vi "GDSLvClass_OpenClass.vi"(1 "ClassToOpen":path, 5 "error in (no error)":errorcluster, 6 "Project/ApplicationRef(If empty, currect active project will be used)":variant) -> (14 "LVClass.Open":refnum<vi>, 19 "error out":errorcluster)   [LabVIEW 2020]
panel:
  in  "App Ref 2":refnum<vi>
  in  "App Refnum 2":refnum<vi>
  in  "Array 2":refnum<vi>[](array[refnum])
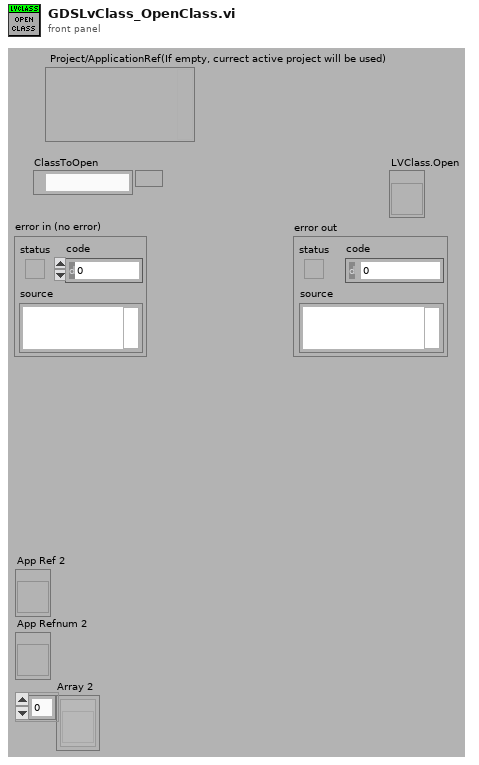
[diagram p1: front panel]
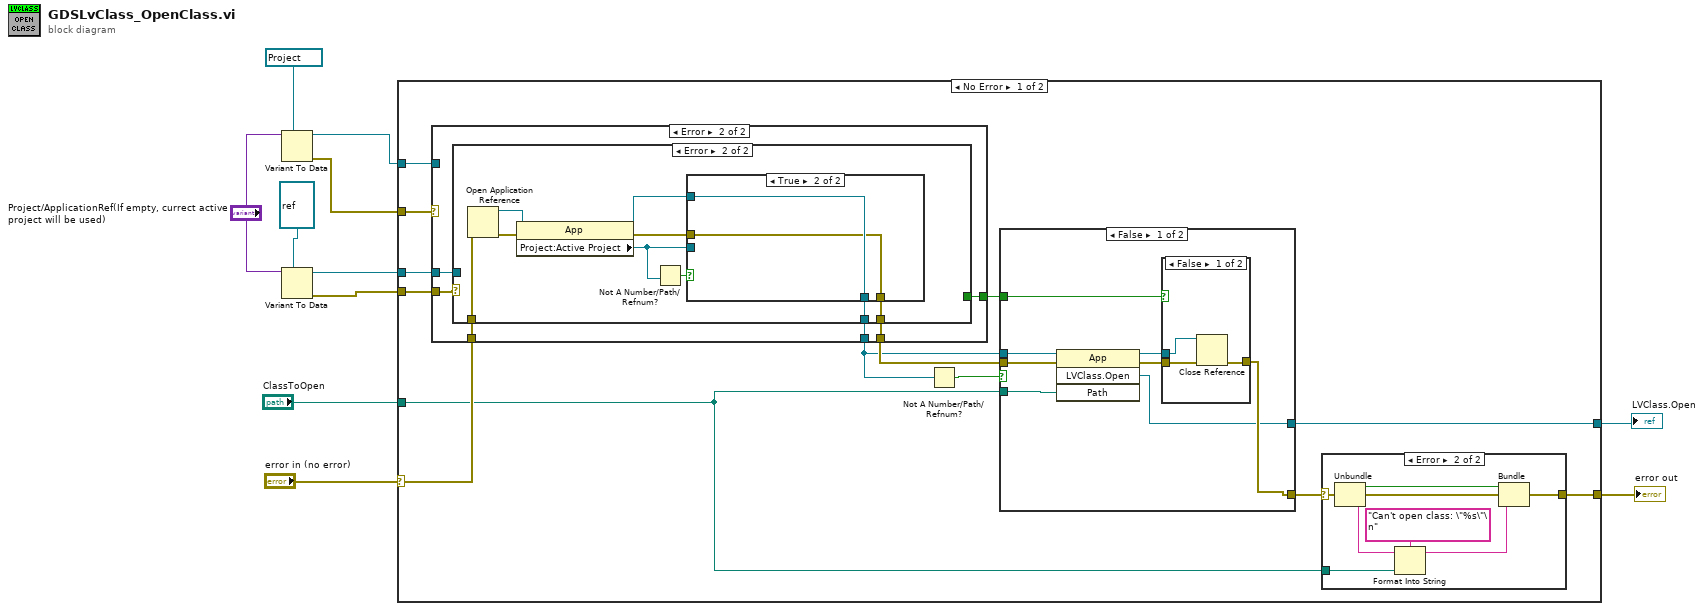
[diagram p0: block diagram]
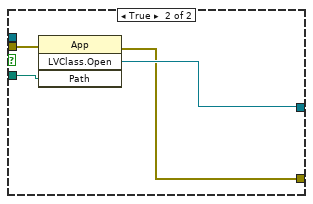
[diagram p4: hidden frame]
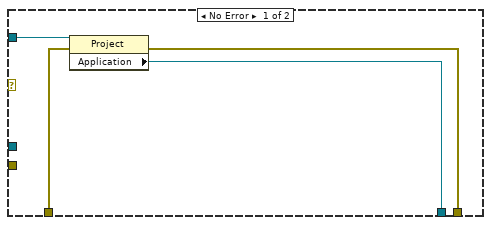
[diagram p5: hidden frame]
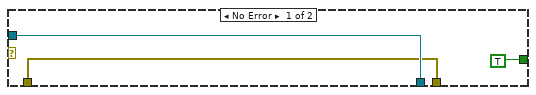
[diagram p6: hidden frame]
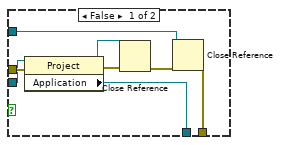
[diagram p7: hidden frame]
diagram:
  n1 = Variant To Data(type=refnum<vi> refnum ("Project/ApplicationRef(If empty, currect active project will be used)"), Variant="Project/ApplicationRef(If empty, currect active project will be used)") -> (data=w3:refnum<vi>, error out=w4:errorcluster)  [unwired: 1 in]
  n2 = Variant To Data(type=refnum<vi> refnum ("application reference"), Variant="Project/ApplicationRef(If empty, currect active project will be used)") -> (data=w1:refnum<vi>, error out=w2:errorcluster)  [unwired: 1 in]
  n3 = case shown="No Error" "error in (no error)" {
    selector: "error in (no error)" -> [w24 w82]
    tunnel: [w12 w82] -> w11
    tunnel: "ClassToOpen" -> [w13 _]
    tunnel: [w22 _] -> w8
    tunnel: w4 -> [w21 _]
    tunnel: w3 -> [w20 _]
    tunnel: w2 -> [w19 _]
    tunnel: w1 -> [w18 _]
    frame No Error {
      n4 = case shown="Error" w21 {
        tunnel: w24 -> [w52 w59]
        tunnel: [w50 w58] -> w16
        tunnel: [w51 w57] -> w23
        tunnel: w20 -> [w53 _]
        tunnel: w19 -> [_ w56]
        tunnel: w18 -> [_ w55]
        tunnel: [_ w54] -> w17
        frame No Error {
          n5 = property class="Project"(reference=w53, error in=w52) -> (error out=w51:errorcluster, "Application"=w50:refnum<vi>)  [unwired: 1 out]
        }
        frame Error {
          n6 = case shown="Error" w56 {
            tunnel: w59 -> [w61 w71]
            tunnel: [w62 w66] -> w58
            tunnel: [w61 w65] -> w57
            tunnel: w55 -> [w62 _]
            tunnel: [TRUE _] -> w54
            frame No Error {
            }
            frame Error {
              n7 = Open Application Reference(8:w71) -> (0:w70:errorcluster, 3:w69:refnum<vi>)  [unwired: 3 in]
              n8 = property class="App"(reference=w69, error in=w70) -> (reference out=w67:refnum<vi>, error out=w68:errorcluster, "Project:Active Project"=w64:refnum<vi>)
              n9 = Not A Number/Path/Refnum?(number/path/refnum=w64) -> (NaN/Path/Refnum?=w63:bool)
              n10 = case shown="True" w63 {
                tunnel: w68 -> [w79 w80]
                tunnel: w67 -> [w78 w81]
                tunnel: [w77 w81] -> w66
                tunnel: [w76 w80] -> w65
                tunnel: w64 -> [w75 _]
                frame False {
                  n11 = property class="Project"(reference=w75, error in=w79) -> (reference out=w73:refnum<vi>, error out=w74:errorcluster, "Application"=w77:refnum<vi>)
                  n12 = Close Reference(reference=w73, error in (no error)=w74) -> (error out=w72:errorcluster)
                  n13 = Close Reference(reference=w78, error in (no error)=w72) -> (error out=w76:errorcluster)
                }
                frame True {
                }
              }
            }
          }
        }
      }
      n14 = Not A Number/Path/Refnum?(number/path/refnum=w16) -> (NaN/Path/Refnum?=w15:bool)
      n15 = case shown="False" w15 {
        tunnel: w13 -> [w41 w48]
        tunnel: w23 -> [w40 w49]
        tunnel: [w37 w46] -> w14
        tunnel: [w36 w47] -> w22
        tunnel: w17 -> [w35 _]
        tunnel: w16 -> [w34 _]
        frame False {
          n16 = invoke class="App" method="LVClass.Open"(reference=w34, error in=w40, "Path"=w41) -> (reference out=w38:refnum<vi>, error out=w39:errorcluster, "LVClass.Open"=w36:refnum<vi>)  [unwired: 1 in, 1 out]
          n17 = case shown="False" w35 {
            tunnel: w39 -> [w44 w45]
            tunnel: w38 -> [w43 _]
            tunnel: [w42 w45] -> w37
            frame False {
              n18 = Close Reference(reference=w43, error in (no error)=w44) -> (error out=w42:errorcluster)
            }
            frame True {
            }
          }
        }
        frame True {
          n19 = invoke class="App" method="LVClass.Open"(error in=w49, "Path"=w48) -> (error out=w46:errorcluster, "LVClass.Open"=w47:refnum<vi>)  [unwired: 2 in, 2 out]
        }
      }
      n20 = case shown="Error" w14 {
        selector: w14 -> [w25 w30]
        tunnel: w13 -> [_ w32]
        tunnel: [w25 w29] -> w12
        frame No Error {
        }
        frame Error {
          n21 = Unbundle(w30) -> ("status"=w27:bool, "code"=w26:i32, "source"=w31:string)
          n22 = Format Into String(format string="Can't open class: \"%s\"\n", initial string=w31, w32) -> (resulting string=w28:string)  [unwired: 1 in, 1 out]
          n23 = Bundle(cluster=w30, "status"=w27, "code"=w26, "source"=w28) -> (w29:errorcluster)
        }
      }
    }
    frame Error {
      (unwired) string[] []
      (unwired) "" ("Name")
      (unwired) FALSE
    }
  }
  "error out" <- w11
  "LVClass.Open" <- w8
